vi "Manual Override Button Enable Disable Shared.vi"(0 "Stop Program":refnum<vi>, 1 "Valves on Shared Lines":i32, 2 "Pump Shared Lock Claimed Array":refnum<vi>, 3 "Shared Manual Valve Array":refnum<vi>) -> ()   [LabVIEW 2022 SP3]
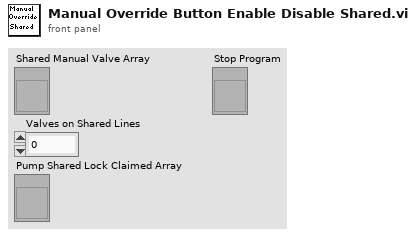
[diagram p1: front panel]
types:
  T1 = enum8{"Enabled", "Disabled", "Disabled and Grayed Out"}
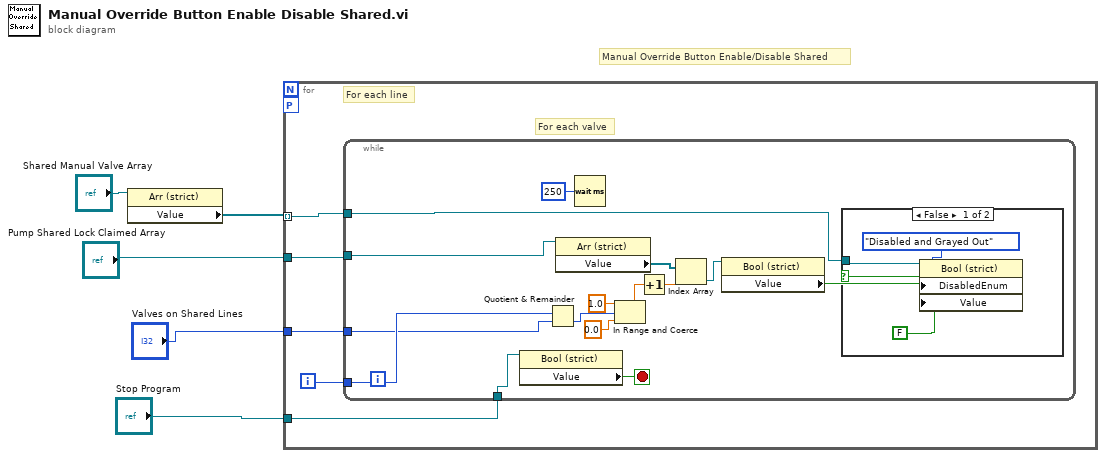
[diagram p0: block diagram]
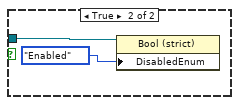
[diagram p2: hidden frame]
diagram:
  # "Manual Override Button Enable/Disable Shared"
  n1 = property class="Arr (strict)"(reference="Shared Manual Valve Array") -> ("Value"=w5:refnum<vi>[])  [unwired: 1 in, 2 out]
  n2 = for {
    tunnel: w5 -> [w10] mode=indexing
    workers-P: _ -> [_]
    tunnel: "Valves on Shared Lines" -> [w8]
    tunnel: "Pump Shared Lock Claimed Array" -> [w7]
    tunnel: "Stop Program" -> [w6]
    i -> [w9]
    # "For each valve"
    # "For each line"
    n3 = while {
      tunnel: w10 -> [w25]
      tunnel: w9 -> [w16]
      tunnel: w8 -> [w14]
      tunnel: w7 -> [w13]
      tunnel: w6 -> [w11]
      stop <- w12 stop-if-true
      n4 = property class="Bool (strict)"(reference=w11) -> ("Value"=w12:bool)  [unwired: 1 in, 2 out]
      n5 = Quotient & Remainder(x=w16, y=w14) -> (floor(x/y)=w15:i32)  [unwired: 1 out]
      n6 = property class="Arr (strict)"(reference=w13) -> ("Value"=w23:refnum<vi>[])  [unwired: 1 in, 2 out]
      n7 = Wait (ms)(milliseconds to wait=u32 250 ("millisecond multiple")) -> ()  [unwired: 1 out]
      n8 = In Range and Coerce(upper limit=1.0, x=w15, lower limit=0.0) -> (coerced(x)=w17:dbl)  [unwired: 1 out]
      n9 = Increment(x=w17) -> (x+1=w20:dbl)
      n10 = Index Array(array=w23, index=w20) -> (element=w22:refnum<vi>)
      n11 = property class="Bool (strict)"(reference=w22) -> ("Value"=w21:bool)  [unwired: 1 in, 2 out]
      n12 = case shown="False" w21 {
        tunnel: w25 -> [w28 w29]
        frame False {
          n13 = property class="Bool (strict)"(reference=w28, "DisabledEnum"=T1."Disabled and Grayed Out" ("Disabled"), "Value"=FALSE) -> ()  [unwired: 1 in, 2 out]
        }
        frame True {
          n14 = property class="Bool (strict)"(reference=w29, "DisabledEnum"=T1."Enabled" ("Disabled")) -> ()  [unwired: 1 in, 2 out]
        }
      }
    }
  }
